vi "Create_Item_List.vi"(1 "Running":bool, 2 "Alias Table":string[][](array[string]), 3 "Sequence":cluster{string, string[], dbl[], dbl}[](array[cluster])) -> (0 "Item List":string[](array[string]))   [LabVIEW 2011]
doc: "This VI creates an \"Item List\" which supplies the appropriate values for the graphical user-editable list in the editor. The \"Running\" parameter alters the item to list to make it appropriate for use in Run_Sequence.vi."
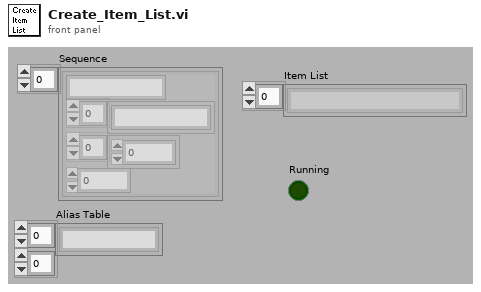
[diagram p1: front panel]
types:
  T1 = enum16{"Discrete", "Continuous", "Instantaneous", "Finite"}
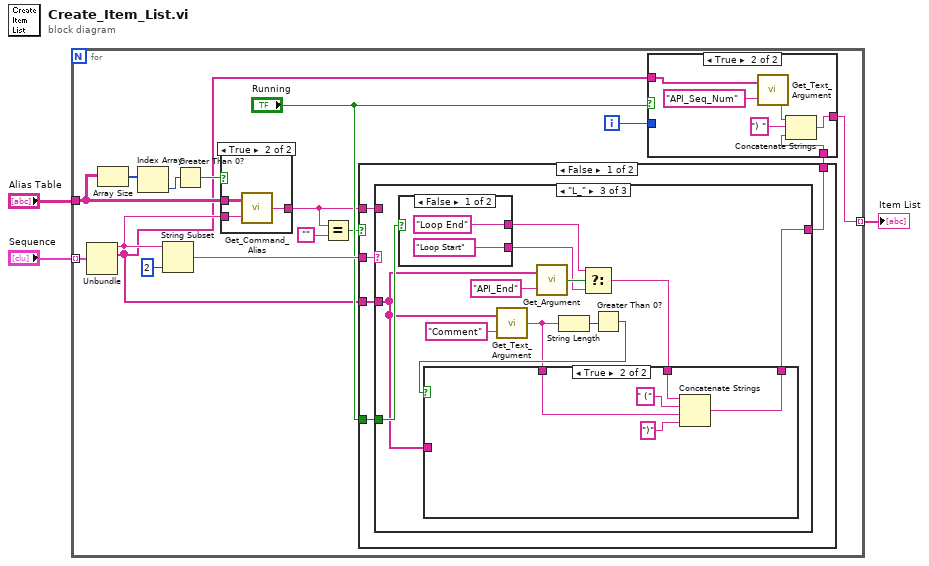
[diagram p0: block diagram]
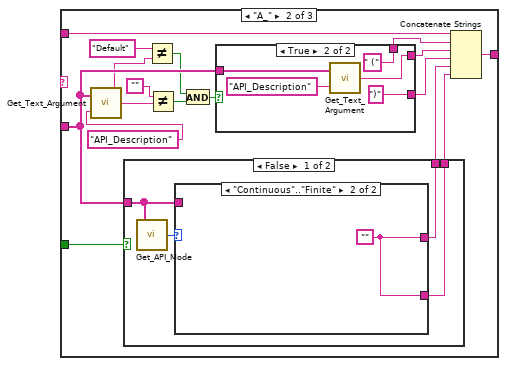
[diagram p3: hidden frame]
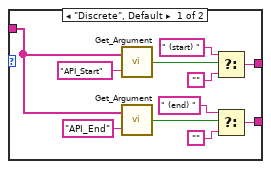
[diagram p4: hidden frame]
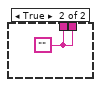
[diagram p5: hidden frame]
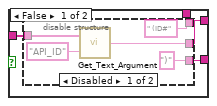
[diagram p6: hidden frame]
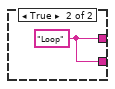
[diagram p8: hidden frame]
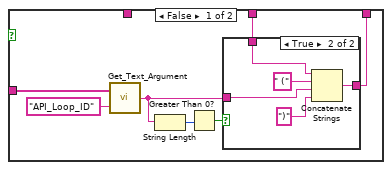
[diagram p9: hidden frame]
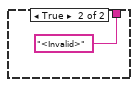
[diagram p11: hidden frame]
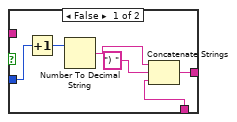
[diagram p12: hidden frame]
diagram:
  n1 = for {
    tunnel: [w19] -> w3 mode=indexing
    tunnel: "Sequence" -> [w18] mode=indexing
    tunnel: "Alias Table" -> [w13]
    i -> [w17]
    n2 = Unbundle(w18) -> (w14:string, w4:string[])  [unwired: 2 out]
    n3 = Array Size(array=w13) -> (size(s)=w12:i32[])
    n4 = Index Array(array=w12) -> (element=w10:i32)  [unwired: 1 in]
    n5 = String Subset(string=w14, length (rest)=2 ("length (rest)")) -> (substring=w9:string)  [unwired: 1 out]
    n6 = Greater Than 0?(x=w10) -> (x > 0?=w11:bool)
    n7 = case shown="True" w11 {
      tunnel: w13 -> [_ w122]
      tunnel: w14 -> [w119 w121]
      tunnel: [w119 w120] -> w6
      frame False {
      }
      frame True {
        n8 = call "Get_Command_Alias.vi"("Command"=w121, "Alias Table"=w122) -> ("Alias"=w120:string)
      }
    }
    n9 = Equal?(x=w6, y="") -> (x = y?=w5:bool)
    n10 = case shown="False" w5 {
      tunnel: w4 -> [w24 _]
      tunnel: [w23 "<Invalid>" ("f")] -> w15
      tunnel: w6 -> [w22 _]
      tunnel: w9 -> [w21 _]
      tunnel: "Running" -> [w20 _]
      frame False {
        n11 = case shown="\"L_\"" w21 {
          tunnel: w24 -> [_ w33 w73]
          tunnel: w22 -> [w25 w40 _]
          tunnel: [w25 w41 w80] -> w23
          tunnel: w20 -> [_ w26 w74]
          frame Default {
          }
          frame "A_" {
            n12 = call "Get_Text_Argument.vi"("Argument"="API_Description", "Argument List"=w33) -> ("Text"=w31:string)
            n13 = case shown="False" w26 {
              tunnel: [w45 w58] -> w38
              tunnel: [w44 w58] -> w37
              tunnel: w33 -> [w43 _]
              frame False {
                n14 = call "Get_API_Mode.vi"("Argument List"=w43) -> ("API Mode"=w42:T1)
                n15 = case shown="\"Continuous\"..\"Finite\"" w42 {
                  tunnel: [w48 w57] -> w45
                  tunnel: [w47 w57] -> w44
                  tunnel: w43 -> [w46 _]
                  frame "Discrete", Default {
                    n16 = call "Get_Argument.vi"("Argument"="API_Start", "Argument List"=w46) -> ("Enabled"=w55:bool)
                    n17 = call "Get_Argument.vi"("Argument"="API_End", "Argument List"=w46) -> ("Enabled"=w51:bool)
                    n18 = Select(t=" (start) ", s=w55, f="") -> (s? t:f=w48:string)
                    n19 = Select(t=" (end) ", s=w51, f="") -> (s? t:f=w47:string)
                  }
                  frame "Continuous".."Finite" {
                    w57 = ""
                  }
                }
              }
              frame True {
                w58 = ""
              }
            }
            n20 = Not Equal?(x="Default", y=w31) -> (x != y?=w28:bool)
            n21 = Not Equal?(x="", y=w31) -> (x != y?=w29:bool)
            n22 = And(x=w28, y=w29) -> (x .and. y?=w27:bool)
            n23 = case shown="True" w27 {
              tunnel: w33 -> [w62 w72]
              tunnel: [w60 w70] -> w39
              tunnel: [w59 ")" ("string")] -> w36
              tunnel: [w61 " (" ("string")] -> w35
              frame False {
                n24 = disable-structure shown="Disabled" {
                  disable-tunnel: w62 -> [w67 _]
                  disable-tunnel: [" (ID#" ("string") _] -> w61
                  disable-tunnel: [w64 _] -> w60
                  disable-tunnel: [")" _] -> w59
                  frame Disabled {
                    n25 = call "Get_Text_Argument.vi"("Argument"="API_ID", "Argument List"=w67) -> ("Text"=w64:string)
                  }
                  frame Enabled {
                  }
                }
              }
              frame True {
                n26 = call "Get_Text_Argument.vi"("Argument"="API_Description", "Argument List"=w72) -> ("Text"=w70:string)
              }
            }
            n27 = Concatenate Strings(w40, w35, w39, w36, w38, w37) -> (w41:string)
          }
          frame "L_" {
            n28 = case shown="False" w74 {
              tunnel: ["Loop End" ("Argument") w87] -> w82
              tunnel: ["Loop Start" ("Argument") w87] -> w81
              frame False {
              }
              frame True {
                w87 = "Loop" ("Argument")
              }
            }
            n29 = call "Get_Text_Argument.vi"("Argument"="Comment", "Argument List"=w73) -> ("Text"=w75:string)
            n30 = call "Get_Argument.vi"("Argument"="API_End", "Argument List"=w73) -> ("Enabled"=w83:bool)
            n31 = String Length(string=w75) -> (length=w77:i32)
            n32 = Select(t=w82, s=w83, f=w81) -> (s? t:f=w79:string)
            n33 = Greater Than 0?(x=w77) -> (x > 0?=w76:bool)
            n34 = case shown="True" w76 {
              tunnel: [w93 w101] -> w80
              tunnel: w79 -> [w90 w104]
              tunnel: w73 -> [w89 _]
              tunnel: w75 -> [_ w105]
              frame False {
                n35 = call "Get_Text_Argument.vi"("Argument"="API_Loop_ID", "Argument List"=w89) -> ("Text"=w88:string)
                n36 = String Length(string=w88) -> (length=w92:i32)
                n37 = Greater Than 0?(x=w92) -> (x > 0?=w91:bool)
                n38 = case shown="True" w91 {
                  tunnel: [w95 w98] -> w93
                  tunnel: w88 -> [_ w97]
                  tunnel: w90 -> [w95 w96]
                  frame False {
                  }
                  frame True {
                    n39 = Concatenate Strings(w96, " (" ("string"), w97, ")" ("string")) -> (w98:string)
                  }
                }
              }
              frame True {
                n40 = Concatenate Strings(w104, " (" ("string"), w105, ")" ("string")) -> (w101:string)
              }
            }
          }
        }
      }
      frame True {
      }
    }
    n41 = case shown="True" "Running" {
      tunnel: [w112 w113] -> w19
      tunnel: w17 -> [w110 _]
      tunnel: w15 -> [w109 w115]
      tunnel: w4 -> [_ w117]
      frame False {
        n42 = Increment(x=w110) -> (x+1=w111:i32)
        n43 = Number To Decimal String(number=w111) -> (decimal integer string=w108:string)  [unwired: 1 out]
        n44 = Concatenate Strings(w108, ") " ("string"), w109) -> (w112:string)
      }
      frame True {
        n45 = call "Get_Text_Argument.vi"("Argument"="API_Seq_Num", "Argument List"=w117) -> ("Text"=w116:string)
        n46 = Concatenate Strings(w116, ") " ("string"), w115) -> (w113:string)
      }
    }
  }
  "Item List" <- w3
